vi "Corner Placer.vi"(1 "Center of Mass":T1={"Numeric Control"=640.0, "Numeric Control"=480.0}, 2 "Point":T1={"Numeric Control"=640.0, "Numeric Control"=480.0}) -> (0 "Index":i8)   [LabVIEW 2011]
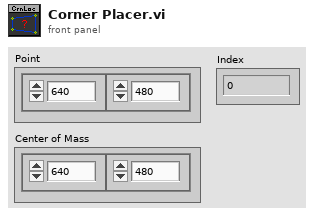
[diagram p1: front panel]
types:
  T1 = cluster{"Numeric Control":dbl, "Numeric Control":dbl}
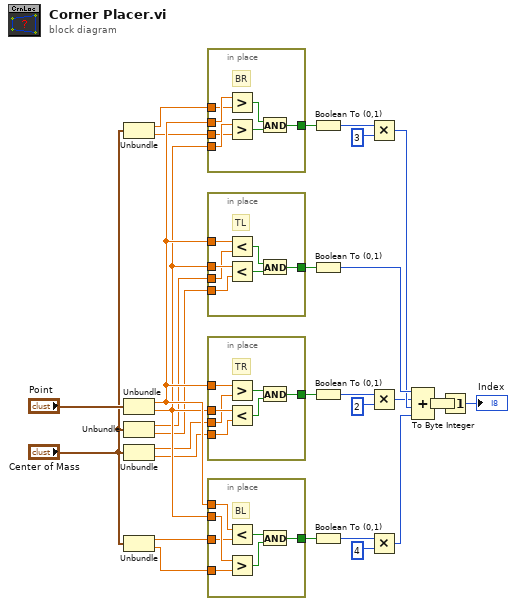
[diagram p0: block diagram]
diagram:
  n1 = Unbundle("Center of Mass") -> ("Numeric Control"=w23:dbl, "Numeric Control"=w22:dbl)
  n2 = Unbundle("Point") -> ("Numeric Control"=w29:dbl, "Numeric Control"=w28:dbl)
  n3 = Unbundle("Center of Mass") -> ("Numeric Control"=w27:dbl, "Numeric Control"=w26:dbl)
  n4 = Unbundle("Center of Mass") -> ("Numeric Control"=w25:dbl, "Numeric Control"=w24:dbl)
  n5 = Unbundle("Center of Mass") -> ("Numeric Control"=w21:dbl, "Numeric Control"=w20:dbl)
  n6 = in-place {
    in-place-border: [w34] -> w17
    in-place-border: w29 -> [w33]
    in-place-border: w28 -> [w32]
    in-place-border: w23 -> [w31]
    in-place-border: w22 -> [w30]
    # "BR"
    n7 = Greater?(x=w33, y=w31) -> (0:w35:bool)
    n8 = Greater?(x=w32, y=w30) -> (0:w36:bool)
    n9 = And(x=w35, y=w36) -> (x .and. y?=w34:bool)
  }
  n10 = in-place {
    in-place-border: [w41] -> w16
    in-place-border: w29 -> [w40]
    in-place-border: w28 -> [w39]
    in-place-border: w27 -> [w38]
    in-place-border: w26 -> [w37]
    # "TL"
    n11 = Less?(x=w40, y=w38) -> (x < y?=w42:bool)
    n12 = Less?(x=w39, y=w37) -> (x < y?=w43:bool)
    n13 = And(x=w42, y=w43) -> (x .and. y?=w41:bool)
  }
  n14 = in-place {
    in-place-border: [w48] -> w15
    in-place-border: w29 -> [w47]
    in-place-border: w28 -> [w46]
    in-place-border: w25 -> [w45]
    in-place-border: w24 -> [w44]
    # "TR"
    n15 = Greater?(x=w47, y=w45) -> (0:w49:bool)
    n16 = Less?(x=w46, y=w44) -> (x < y?=w50:bool)
    n17 = And(x=w49, y=w50) -> (x .and. y?=w48:bool)
  }
  n18 = in-place {
    in-place-border: [w55] -> w14
    in-place-border: w29 -> [w54]
    in-place-border: w28 -> [w53]
    in-place-border: w21 -> [w52]
    in-place-border: w20 -> [w51]
    # "BL"
    n19 = Less?(x=w54, y=w52) -> (x < y?=w56:bool)
    n20 = Greater?(x=w53, y=w51) -> (0:w57:bool)
    n21 = And(x=w56, y=w57) -> (x .and. y?=w55:bool)
  }
  n22 = Boolean To (0,1)(Boolean=w17) -> (0, 1=w12:i16)
  n23 = Boolean To (0,1)(Boolean=w16) -> (0, 1=w13:i16)
  n24 = Boolean To (0,1)(Boolean=w15) -> (0, 1=w6:i16)
  n25 = Boolean To (0,1)(Boolean=w14) -> (0, 1=w3:i16)
  n26 = Multiply(x=w12, y=i16 3) -> (x*y=w9:i16)
  n27 = Multiply(x=w6, y=i16 2) -> (x*y=w7:i16)
  n28 = Multiply(x=w3, y=i16 4) -> (x*y=w4:i16)
  n29 = Compound Arithmetic op=ADD(w13, w7, w9, w4) -> (w11:i16)
  n30 = To Byte Integer(number=w11) -> (8bit integer=w1:i8)
  n31 = Decrement(x=w1) -> (x-1=→"Index":i8)
